vi "Write Number of Tests Sockets.vi"(8 "error in (no error)":errorcluster, 11 "Number of Tests Sockets":u8=1) -> (0 "error out":errorcluster)   [LabVIEW 2019, in "Assert.lvlib"]
uses:
  Assert.lvlib
  f9b623bd-8877-4db9-9b26-c69f2f87cc45.vi
  Unit Test Engine Global.vi
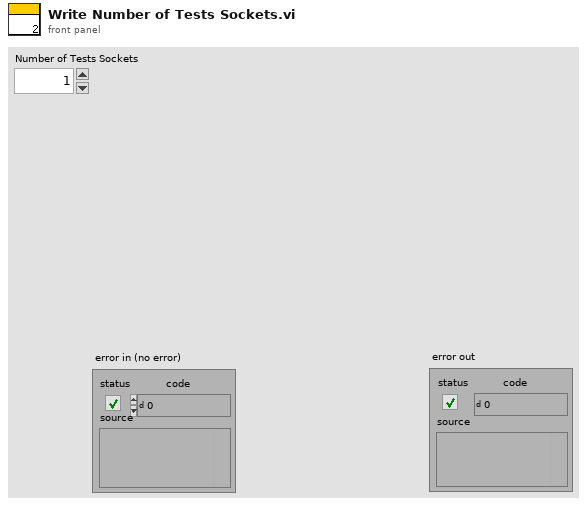
[diagram p1: front panel]
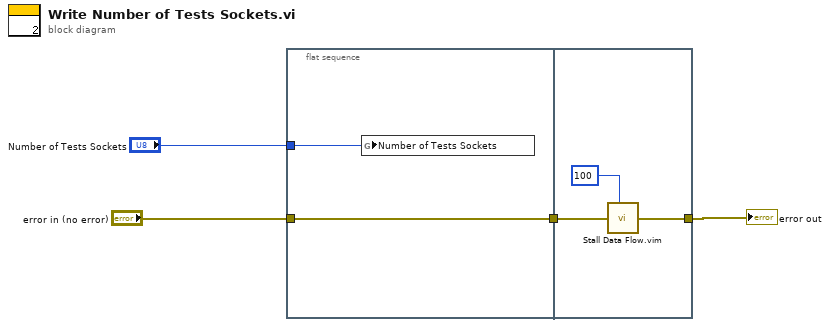
[diagram p0: block diagram]
diagram:
  n1 = flat-sequence {
    tunnel: "Number of Tests Sockets" -> [w6]
    tunnel: [w5] -> w2
    tunnel: "error in (no error)" -> [w5]
    tunnel: [w8] -> w3
    tunnel: w2 -> [w9]
    frame #0 {
      n2 = global write "Unit Test Engine Global.vi" "Number of Tests Sockets"(w6) -> ()
    }
    frame #1 {
      n3 = call "Stall Data Flow.vim"("value in"=w9, "milliseconds to wait"=u32 100) -> ("value out"=w8:errorcluster)  [unwired: 1 out]
    }
  }
  "error out" <- w3
